vi "Check Inspecting Status.vi"(0 "Inspection Limits":T1={"MaxSamples"=50800, "PosToStartScan"=50800, "PosToEndScan"=0, "ScanLength"=50800}, 5 "Status Byte":u16, 9 "Loop Counter":i32, 11 "error in (no error)":errorcluster, 12 "Max Tries":i32) -> (1 "Last Sample No.":u32, 3 "Stop Inspection":bool, 4 "Last Sample":u32[](array[numeric]), 6 "Encoder Count out":i32, 8 "Inside Scan Region":bool, 10 "Success":bool, 14 "DebugLog String":string, 15 "error out":errorcluster)   [LabVIEW 2015, in "Tool Module.lvlib"]
doc: "<b>Note:</b> This VI was modified by the <b>Validate DQMH Module</b> tool to turn off automatic error handling."
uses:
  Tool Module.lvlib
  _Inspection Limits cluster--typedef.ctl
  ToolModGLOB.vi
  <vilib>/Utility/error.llb/Error Cluster From Error Code.vi
  <vilib>/ErrorRing/Error Ring.xnode
  Tool Config/Tool Cfg.lvlib
  Tool Interface/Tool Interface.lvlib
panel:
  out "Probe Data":u32[](array[numeric])
  # "(-1: ignore loop count)"
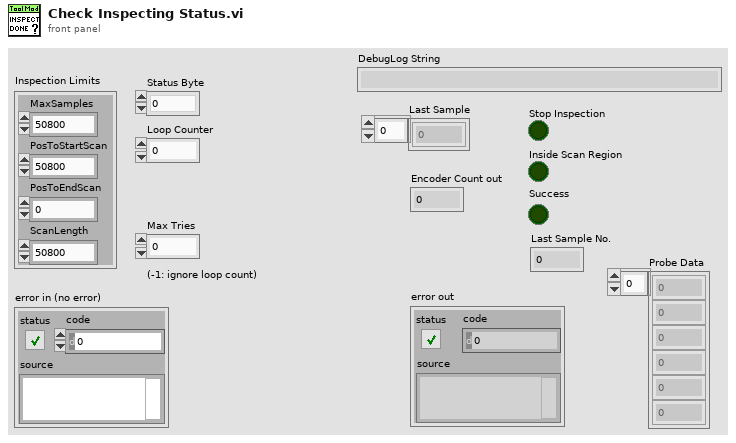
[diagram p1: front panel]
types:
  T1 = typedef "Tool Module.lvlib/_Inspection Limits cluster--typedef.ctl" = cluster{"MaxSamples":i32, "PosToStartScan":i32, "PosToEndScan":i32, "ScanLength":i32}
  T2 = typedef "_Data Stream Fmt Params Cluster--typedef.ctl" = cluster{"Samples per Block":i32, "Raw Data Status Len":i32, "Fltr Data Status Len":i32}
  T3 = typedef "Tool Cfg.lvlib/_Tool Operation Config Cluster--typedef.ctl" = cluster{"Use Tool Cfg":bool, "Use Tool Cal":bool, "Fake Data?":bool, "Mode":i16, "Array Subset Length":i16, "nArrays to Read":i16, "Full Array Read Length":i16, "nSubarrays/Sensor":i16}
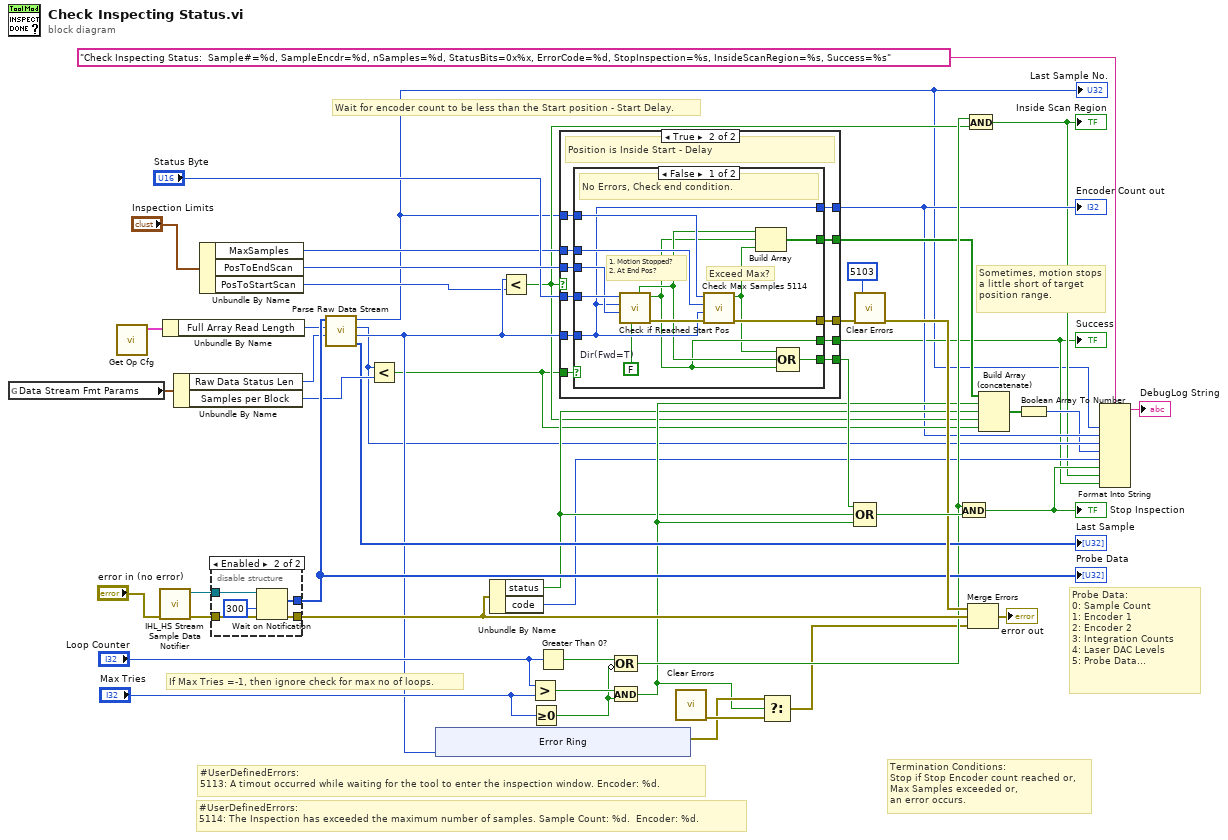
[diagram p0: block diagram]
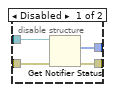
[diagram p2: hidden frame]
diagram:
  # "If Max Tries =-1, then ignore check for max no of loops."
  # "#UserDefinedErrors:\n5113: A timout occurred while waiting for the tool to enter the inspection window. Encoder: %d."
  # "Wait for encoder count to be less than the Start position - Start Delay."
  # "#UserDefinedErrors:\n5114: The Inspection has exceeded the maximum number of samples. Sample Count: %d.  Encoder: %d."
  # "Probe Data:\n0: Sample Count\n1: Encoder 1\n2: Encoder 2\n3: Integration Counts\n4: Laser DAC Levels\n5: Probe Data..."
  # "Sometimes, motion stops a little short of target position range."
  # "Termination Conditions:\nStop if Stop Encoder count reached or,\nMax Samples exceeded or,\nan error occurs."
  n1 = global read "ToolModGLOB.vi" "Data Stream Fmt Params"() -> (w35:T2)
  n2 = call "Get Op Cfg.vi"() -> ("Tool Operation Config"=w36:T3)  [unwired: 11 in]
  n3 = call "IHL_HS Stream Sample Data Notifier.vi"("error in (no error)"="error in (no error)") -> ("error out"=w45:errorcluster, "Sample Data notifier out"=w1:refnum<notifier>)  [unwired: 9 in]
  n4 = Unbundle By Name(w36) -> ("Full Array Read Length"=w33:i16)
  n5 = Unbundle By Name(w35) -> ("Raw Data Status Len"=w34:i32, "Samples per Block"=w32:i32)
  n6 = Unbundle By Name("Inspection Limits") -> ("MaxSamples"=w31:i32, "PosToEndScan"=w39:i32, "PosToStartScan"=w18:i32)
  n7 = disable-structure shown="Enabled" {
    disable-tunnel: w1 -> [w52 w55]
    disable-tunnel: [w51 w57] -> w26
    disable-tunnel: w45 -> [w50 w56]
    disable-tunnel: [w49 w54] -> w38
    frame Disabled {
      n8 = Get Notifier Status(notifier=w52, error in (no error)=w50) -> (current notification=w49:u32[], error out=w51:errorcluster)  [unwired: 3 out]
    }
    frame Enabled {
      n9 = Wait on Notification(notifier=w55, timeout in ms (-1)=300, error in (no error)=w56) -> (notification=w54:u32[], error out=w57:errorcluster)  [unwired: 1 in, 2 out]
    }
  }
  "Probe Data" <- w38
  n10 = call "Parse Raw Data Stream.vi"("Status Hdr Length"=w34, "Pixel Array Length"=w33, "Sample Data Array"=w38) -> ("Last Sample"=→"Last Sample":u32[], "Encoder Out"=w24:i32, "nSamples"=w10:u32, "Last Sample No."=w2:u32)  [unwired: 4 in, 1 out]
  "Last Sample No." <- w2
  n11 = Less?(x=w10, y=w32) -> (x < y?=w13:bool)
  n12 = xnode "Error Ring"("parameter 0"=w24) -> ("error out"=w21:errorcluster)
  n13 = Unbundle By Name(w26) -> ("status"=w15:bool, "code"=w7:i32)
  n14 = Less?(x=w24, y=w18) -> (x < y?=w14:bool)
  n15 = Greater?(x="Loop Counter", y="Max Tries") -> (0:w27:bool)
  n16 = Greater Or Equal To 0?(x="Max Tries") -> (x >= 0?=w19:bool)
  n17 = Greater Than 0?(x="Loop Counter") -> (x > 0?=w29:bool)
  n18 = case shown="True" w14 {
    tunnel: w13 -> [_ w69]
    tunnel: w2 -> [_ w66]
    tunnel: [_ w68] -> w48
    tunnel: w24 -> [w58 w64]
    tunnel: [w58 w67] -> w11
    tunnel: "Status Byte" -> [_ w65]
    tunnel: w31 -> [_ w63]
    tunnel: [_ w62] -> w43
    tunnel: w39 -> [_ w61]
    tunnel: [_ w60] -> w3
    tunnel: [_ w59] -> w17
    frame False {
      # "Don't check anything if the probe hasn't moved the start delay length  yet."
    }
    frame True {
      # "Position is Inside Start - Delay"
      n19 = case shown="False" w69 {
        tunnel: [w75 w83] -> w67
        tunnel: w64 -> [w75 w83]
        tunnel: [w78 _] -> w68
        tunnel: w66 -> [w82 _]
        tunnel: w65 -> [w77 _]
        tunnel: w63 -> [w81 _]
        tunnel: [w79 _] -> w62
        tunnel: w61 -> [w76 _]
        tunnel: [w72 _] -> w60
        tunnel: [w70 _] -> w59
        frame False {
          w74 = FALSE  # Dir(Fwd=T)
          # "1. Motion Stopped?\n2. At End Pos?"
          # "Exceed Max?"
          # "No Errors, Check end condition."
          n20 = call "Check if Reached Start Pos.vi"("Dir(Fwd=T)"=w74, "Target Encdr Pos."=w76, "Cur Encoder Value"=w75, "Status Byte"=w77) -> ("error out"=w80:errorcluster, "ReachedPos?"=w72:bool, "MotionStopped?"=w73:bool)  [unwired: 3 in, 2 out]
          n21 = call "Check Max Samples 5114.vi"("error in (no error)"=w80, "Encoder"=w75, "Max Samples"=w81, "Sample Count"=w82) -> ("error out"=w79:errorcluster, "Exceed Max?"=w71:bool)  [unwired: 6 in]
          n22 = Build Array(w73, w72, w71) -> (w70:bool[])
          n23 = Compound Arithmetic op=OR(w71, w73, w72) -> (w78:bool)
        }
        frame True {
          # "If Partial Array or Timeout, Go around again.\nMain App needs to send cmd to Stop Inspecting to get out of this loop. (or one of the other termination conditions."
        }
      }
    }
  }
  "Encoder Count out" <- w11
  "Success" <- w3
  n24 = And(x=w27, y=w19) -> (x .and. y?=w16:bool)
  n25 = Compound Arithmetic op=OR(w29, invert w19) -> (w23:bool)
  n26 = call <vilib>:"Clear Errors.vi"() -> ("error out"=w22:errorcluster)  [unwired: 6 in, 1 out]
  n27 = Select(t=w21, s=w16, f=w22) -> (s? t:f=w20:errorcluster)
  n28 = Compound Arithmetic op=OR(w48, w15, w16) -> (w47:bool)
  n29 = call <vilib>:"Clear Errors.vi"("error in (no error)"=w43, "specific error code to clear (0: all)"=5103) -> ("error out"=w42:errorcluster)  [unwired: 4 in, 1 out]
  n30 = And(x=w23, y=w47) -> (x .and. y?=w6:bool)
  "Stop Inspection" <- w6
  n31 = And(x=w23, y=w14) -> (x .and. y?=w5:bool)
  "Inside Scan Region" <- w5
  n32 = Merge Errors(w42, w26, w20) -> (→"error out":errorcluster)
  n33 = Build Array (concatenate)(w17, w16, w15, w14, w13) -> (w9:bool[])
  n34 = Boolean Array To Number(Boolean array=w9) -> (number=w8:u32)
  n35 = Format Into String(format string="Check Inspecting Status:  Sample#=%d, SampleEncdr=%d, nSamples=%d, StatusBits=0x%x, ErrorCode=%d, StopInspection=%s, InsideScanRegion=%s, Success=%s", w2, w11, w10, w8, w7, w6, w5, w3) -> (resulting string=→"DebugLog String":string)  [unwired: 2 in, 1 out]
